vi "farmers.vi"() -> ()   [LabVIEW 2013]
panel:
  out "output":cluster{string[][]}[](array[cluster])
  in  "input":cluster{"Array 2":u32[][]}[](array[cluster])=[{"Array 2"=[[1, 5, 2], [2, 4, 7], [3, 6, 9]]}, {"Array 2"=[[1, 0, 2, 5, 8], [2, 3, 4, 7, 9], [3, 5, 7, 8, 9], [1, 2, 5, 4, 2], [3, 3, 5, 2, 1]]}, {"Array 2"=[[0, 2, 1, 3], [2, 1, 0, 4], [3, 3, 3, 3], [5, 5, 2, 1]]}]
  # "A A B\nA A B\nA A A"
  # "A A A A A\nA A A A A\nB B A C C\nB B B C C\nB B C C C"
  # "A A B B\nA B B B\nA B B C\nA C C C"
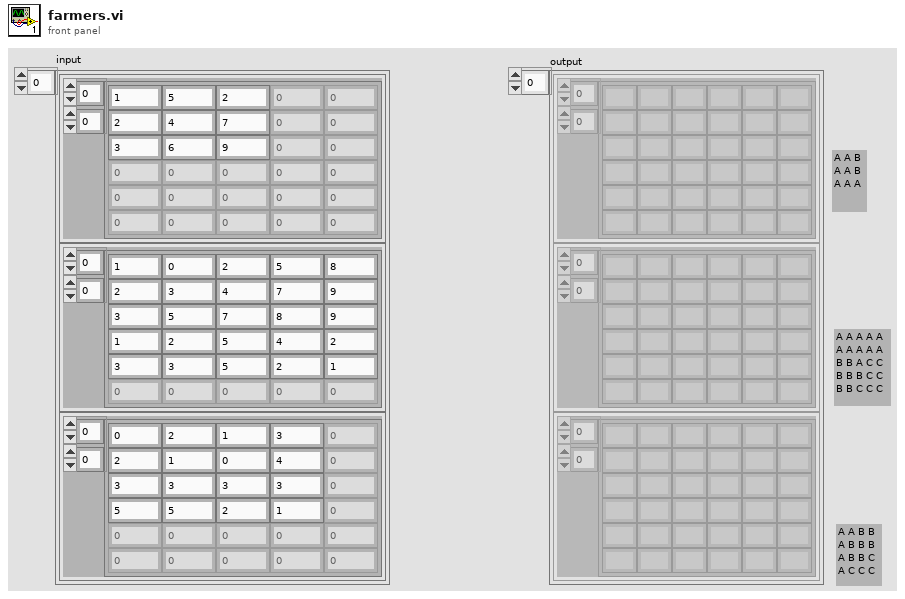
[diagram p1: front panel]
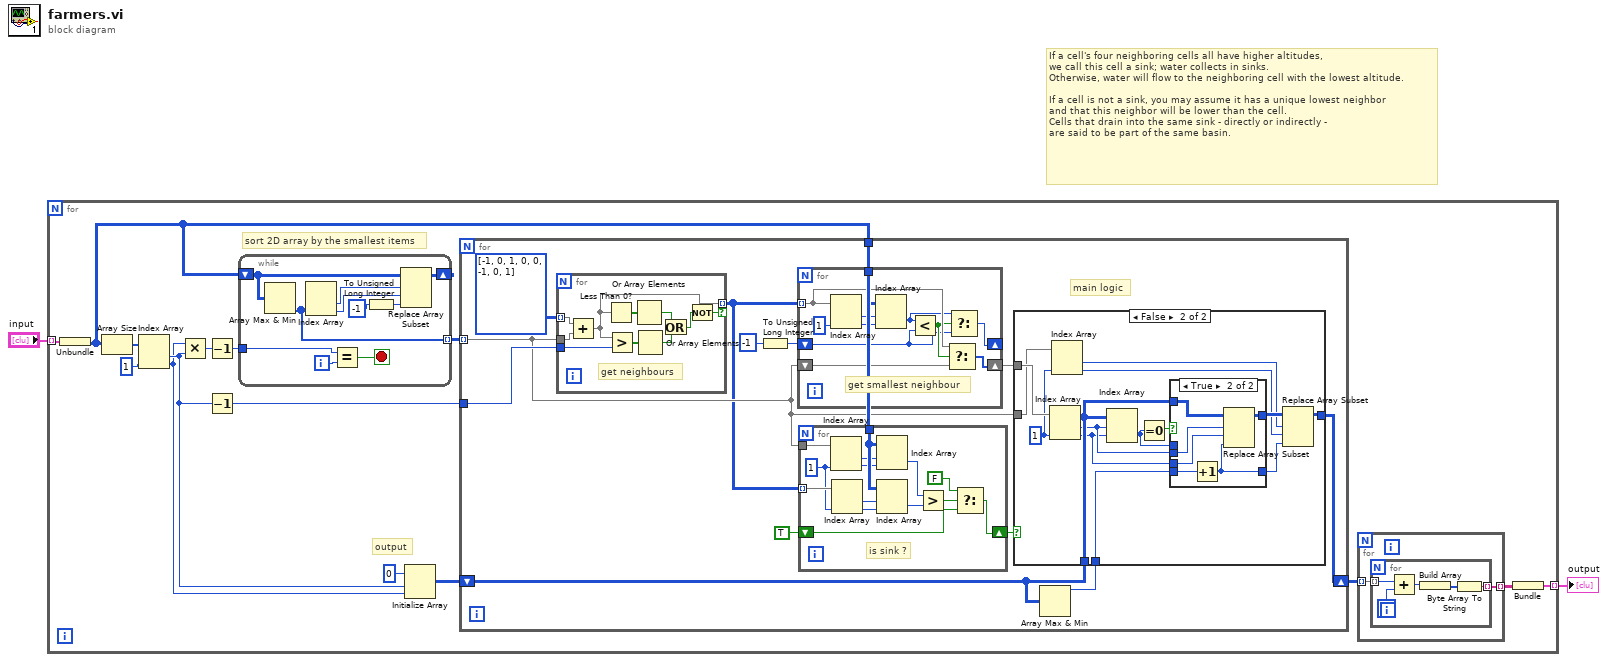
[diagram p0: block diagram]
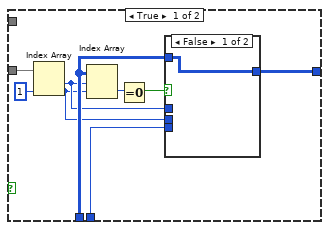
[diagram p2: hidden frame]
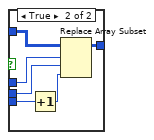
[diagram p3: hidden frame]
diagram:
  # "If a cell's four neighboring cells all have higher altitudes, \nwe call this cell a sink; water collects in sinks.\nOtherwise, water will flow to the neighboring cell with the lowest altitude.\n\nIf a cell is not a sink, you may assume it has a unique lowest neighbor \nand that this neighbor will be lower than the cell.\nCells that drain into the same sink - directly or indirectly - \nare said to be part of the same basin."
  n1 = for {
    tunnel: "input" -> [w7] mode=indexing
    tunnel: [w5] -> w1 mode=indexing
    # "output"
    # "sort 2D array by the smallest items"
    n2 = Unbundle(w7) -> ("Array 2"=w6:u32[][])
    n3 = Array Size(array=w6) -> (size(s)=w17:i32[])
    n4 = Index Array(array=w17, index #2=1 ("index")) -> (element #1=w10:i32, element #2=w9:i32)  [unwired: 1 in]
    n5 = Multiply(x=w9, y=w10) -> (x*y=w14:i32)
    n6 = Decrement(x=w14) -> (x-1=w15:i32)
    n7 = Decrement(x=w10) -> (x-1=w13:i32)
    n8 = while {
      shift-right: [w114] -> _
      shift-left: w6 -> [w120]
      tunnel: [w113] -> w12 mode=indexing
      tunnel: w15 -> [w116]
      i -> [w117]
      stop <- w115 stop-if-true
      n9 = Array Max & Min(array=w120) -> (min index (indices)=w113:i32[])  [unwired: 3 out]
      n10 = Index Array(array=w113) -> (element #1=w119:i32, element #2=w118:i32)  [unwired: 2 in]
      n11 = Equal?(x=w116, y=w117) -> (x = y?=w115:bool)
      n12 = To Unsigned Long Integer(number=-1) -> (unsigned 32bit integer=w111:u32)
      n13 = Replace Array Subset(array=w120, new element=w111, index (row)=w119, index (col)=w118) -> (w114:u32[][])
    }
    n14 = Initialize Array(u8 0 ("element"), w10, w9) -> (w8:u8[][])
    n15 = for {
      tunnel: w12 -> [w32] mode=indexing
      tunnel: w13 -> [w36]
      tunnel: w6 -> [w35]
      shift-right: [w29] -> w4
      shift-left: w8 -> [w31]
      # "main logic"
      n16 = for {
        tunnel: w32 -> [w110]
        tunnel: i32[][] [[-1, 0], [1, 0], [0, -1], [0, 1]] -> [w109] mode=indexing
        tunnel: [w106] -> w27 mode=indexing if=w107
        tunnel: w36 -> [w105]
        # "get neighbours"
        n17 = Add(x=w109, y=w110) -> (x+y=w106:i32[])
        n18 = Less Than 0?(x=w106) -> (x < 0?=w108:bool[])
        n19 = Greater?(x=w106, y=w105) -> (0:w104:bool[])
        n20 = Or Array Elements(Boolean array=w108) -> (logical OR=w103:bool)
        n21 = Or Array Elements(Boolean array=w104) -> (logical OR=w102:bool)
        n22 = Or(x=w103, y=w102) -> (x .or. y?=w101:bool)
        n23 = Not(x=w101) -> (.not. x?=w107:bool)
      }
      n24 = To Unsigned Long Integer(number=-1) -> (unsigned 32bit integer=w26:u32)
      n25 = for {
        tunnel: w27 -> [w96] mode=indexing
        tunnel: w35 -> [w100]
        shift-right: [w94] -> w28
        shift-left: w32 -> [w95]
        shift-right: [w93] -> _
        shift-left: w26 -> [w90]
        # "get smallest neighbour"
        n26 = Index Array(array=w96, index #2=1 ("index")) -> (element #1=w98:i32, element #2=w97:i32)  [unwired: 1 in]
        n27 = Index Array(array=w100, index (row)=w98, index (col)=w97) -> (element=w91:u32)
        n28 = Less?(x=w91, y=w90) -> (x < y?=w92:bool)
        n29 = Select(t=w96, s=w92, f=w95) -> (s? t:f=w94:i32[])
        n30 = Select(t=w91, s=w92, f=w90) -> (s? t:f=w93:u32)
      }
      n31 = for {
        tunnel: w27 -> [w86] mode=indexing
        tunnel: w35 -> [w80]
        shift-right: [w84] -> w33
        shift-left: TRUE -> [w85]
        tunnel: w32 -> [w81]
        w82 = 1 ("index")
        # "is sink ?"
        n32 = Index Array(array=w81, index #2=w82) -> (element #1=w79:i32, element #2=w78:i32)  [unwired: 1 in]
        n33 = Index Array(array=w86, index #2=w82) -> (element #1=w89:i32, element #2=w88:i32)  [unwired: 1 in]
        n34 = Index Array(array=w80, index (row)=w79, index (col)=w78) -> (element=w77:u32)
        n35 = Index Array(array=w80, index (row)=w89, index (col)=w88) -> (element=w76:u32)
        n36 = Greater?(x=w77, y=w76) -> (0:w87:bool)
        n37 = Select(t=FALSE, s=w87, f=w85) -> (s? t:f=w84:bool)
      }
      n38 = Array Max & Min(array=w31) -> (max value=w30:u8)  [unwired: 3 out]
      n39 = case shown="False" w33 {
        tunnel: w31 -> [w43 w67]
        tunnel: w32 -> [w46 w59]
        tunnel: w30 -> [w40 w64]
        tunnel: [w39 w61] -> w29
        tunnel: w28 -> [_ w63]
        frame True {
          n40 = Index Array(array=w46, index #2=1 ("index")) -> (element #1=w42:i32, element #2=w41:i32)  [unwired: 1 in]
          n41 = Index Array(array=w43, index (row)=w42, index (col)=w41) -> (element=w44:u8)
          n42 = Equal To 0?(x=w44) -> (x = 0?=w38:bool)
          n43 = case shown="False" w38 {
            tunnel: w43 -> [w47 w53]
            tunnel: w42 -> [_ w52]
            tunnel: w41 -> [_ w51]
            tunnel: w40 -> [_ w50]
            tunnel: [w47 w49] -> w39
            frame False {
            }
            frame True {
              n44 = Increment(x=w50) -> (x+1=w48:u8)
              n45 = Replace Array Subset(array=w53, new element=w48, index (row)=w52, index (col)=w51) -> (w49:u8[][])
            }
          }
        }
        frame False {
          w58 = 1 ("index")
          n46 = Index Array(array=w63, index #2=w58) -> (element #1=w66:i32, element #2=w65:i32)  [unwired: 1 in]
          n47 = Index Array(array=w59, index #2=w58) -> (element #1=w57:i32, element #2=w56:i32)  [unwired: 1 in]
          n48 = Index Array(array=w67, index (row)=w66, index (col)=w65) -> (element=w54:u8)
          n49 = Equal To 0?(x=w54) -> (x = 0?=w62:bool)
          n50 = case shown="True" w62 {
            tunnel: w67 -> [w69 w75]
            tunnel: w66 -> [_ w74]
            tunnel: w65 -> [_ w73]
            tunnel: w64 -> [_ w72]
            tunnel: [w69 w71] -> w60
            tunnel: [w68 w70] -> w55
            tunnel: w54 -> [w68 _]
            frame False {
            }
            frame True {
              n51 = Increment(x=w72) -> (x+1=w70:u8)
              n52 = Replace Array Subset(array=w75, new element=w70, index (row)=w74, index (col)=w73) -> (w71:u8[][])
            }
          }
          n53 = Replace Array Subset(array=w60, new element=w55, index (row)=w57, index (col)=w56) -> (w61:u8[][])
        }
      }
    }
    n54 = for {
      tunnel: w4 -> [w19] mode=indexing
      tunnel: [w18] -> w3 mode=indexing
      n55 = for {
        tunnel: w19 -> [w23] mode=indexing
        tunnel: [w20] -> w18 mode=indexing
        n56 = Add(x=w23, y=u8 64) -> (x+y=w21:u8)
        n57 = Build Array(w21) -> (w24:u8[])
        n58 = Byte Array To String(unsigned byte array=w24) -> (string=w20:string)
      }
    }
    n59 = Bundle(w3) -> (w5:cluster{string[][]})  [unwired: 1 in]
  }
  "output" <- w1
